vi "Drive Finish.vi"   [LabVIEW 2016]
uses:
  <vilib>/Rock Robotics/WPI/Ultrasonic/WPI_UltrasonicRangeUnits.ctl
  <vilib>/Rock Robotics/WPI/Utilities/WPI_GetSetVariantRefNum.vi
  <vilib>/Rock Robotics/WPI/Ultrasonic/WPI_SonarSRF04DigitalRefNum Registry Get.vi
  <vilib>/Rock Robotics/WPI/Ultrasonic/WPI_SonarSRF04DigitalClose.vi
types:
  T1 = typedef "WPI_UltrasonicRangeUnits.ctl" = enum16{"inches", "mm"}
  T2 = typedef "WPI_SolenoidDevRef.ctl" = cluster{"DevStatus":errorcluster, "Pneumatics Control Module":u8, "Forward Solenoid Channel":T3, "Reverse Solenoid Channel":T3}
  T3 = typedef "WPI_SolenoidChannel.ctl" = enum8{"Solenoid 0", "Solenoid 1", "Solenoid 2", "Solenoid 3", "Solenoid 4", "Solenoid 5", "Solenoid 6", "Solenoid 7", "Invalid"}
  T4 = typedef "WPI_JoystickDevRef.ctl" = cluster{"Device":T5}
  T5 = typedef "WPI_JoystickDeviceEnum.ctl" = enum16{"USB 0", "USB 1", "USB 2", "USB 3", "USB 4", "USB 5"}
  T6 = typedef "WPI_RobotDriveDevRef.ctl" = cluster{"DevStatus":errorcluster, "Motors[]":T7[], "Square Inputs":bool, "Max Output":dbl}
  T7 = typedef "WPI_MotorControlDeviceRef.ctl" = cluster{"DeviceStatus":errorcluster, "Type":T8, "PWM":cluster{"PWM Channel":T9, "DeadBand":T10}, "CAN":cluster{"Device Number":u8, "SetOutput VI Ref":variant, "GetOutput VI Ref":variant, "Enable VI Ref":variant, "Disable VI Ref":variant, "Data":variant}, "Invert":bool}
  T8 = typedef "WPI_MotorControlType.ctl" = enum16{"PWM", "CAN"}
  T9 = typedef "FPGA_DIOPWMChannel.ctl" = enum8{"PWM 0", "PWM 1", "PWM 2", "PWM 3", "PWM 4", "PWM 5", "PWM 6", "PWM 7", "PWM 8", "PWM 9", "PWM MXP 0", "PWM MXP 1", "PWM MXP 2", "PWM MXP 3", "PWM MXP 4", "PWM MXP 5", "PWM MXP 6", "PWM MXP 7", "PWM MXP 8", "PWM MXP 9", "Invalid"}
  T10 = typedef "WPI_PWMDeadband.ctl" = cluster{"Name":string, "maxPositivePwm":i32, "minPositivePwm":i32, "centerPwm":i32, "maxNegativePwm":i32, "minNegativePwm":i32, "angularRange":u16}
  T11 = typedef "WPI_CompressorDevRef.ctl" = cluster{"DevStatus":errorcluster, "Pneumatics Control Module":u8}
  T12 = typedef "WPI_EncoderDevRef.ctl" = cluster{"DevStatus":errorcluster, "EncoderIndex":T13, "CounterIndex":T14, "DistancePerCount":dbl, "Decoding Type":T15}
  T13 = typedef "FPGA_EncoderIdx.ctl" = enum8{"Enc 0", "Enc 1", "Enc 2", "Enc 3", "Enc 4", "Enc 5", "Enc 6", "Enc 7", "Invalid"}
  T14 = typedef "FPGA_CounterCtrSystemIndex.ctl" = enum8{"Ctr 0", "Ctr 1", "Ctr 2", "Ctr 3", "Ctr 4", "Ctr 5", "Ctr 6", "Ctr 7", "Invalid"}
  T15 = typedef "WPI_EncoderType.ctl" = enum16{"1x", "2x", "4x"}
  T16 = typedef "WPI_UltrasonicDeviceRef.ctl" = cluster{"DevStatus":errorcluster, "Ping Channel":T17, "Echo Channel":T17, "CntIndex":T14}
  T17 = typedef "FPGA_DIOChannel.ctl" = enum8{"DIO 0", "DIO 1", "DIO 2", "DIO 3", "DIO 4", "DIO 5", "DIO 6", "DIO 7", "DIO 8", "DIO 9", "DIO MXP 0", "DIO MXP 1", "DIO MXP 2", "DIO MXP 3", "DIO MXP 4", "DIO MXP 5", "DIO MXP 6", "DIO MXP 7", "DIO MXP 8", "DIO MXP 9", "DIO MXP 10", "DIO MXP 11", "DIO MXP 12", "DIO MXP 13", "DIO MXP 14", "DIO MXP 15", "SPI Port CS1", "SPI Port CS2", "SPI Port CS3", "SPI Port MISO", "SPI Port MOSI", "Invalid"}
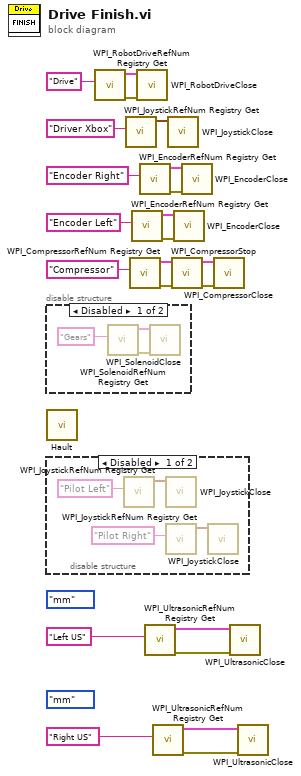
[diagram p0: block diagram]
diagram:
  (unwired) WPI_UltrasonicRangeUnits."mm" ("Range Units")
  (unwired) WPI_UltrasonicRangeUnits."mm" ("Range Units")
  n1 = disable-structure shown="Disabled" {
    frame Disabled {
      n2 = call <vilib>:"WPI_SolenoidRefNum Registry Get.vi"("refnum name"="Gears") -> ("error out"=w24:errorcluster, "SolenoidDevRef"=w25:T2)  [unwired: 9 in]
      n3 = call <vilib>:"WPI_SolenoidClose.vi"("error in (no error)"=w24, "SolenoidDevRef"=w25) -> ()  [unwired: 9 in, 1 out]
    }
    frame Enabled {
    }
  }
  n4 = call <vilib>:"Hault.vi"() -> ()  [unwired: 12 in]
  n5 = disable-structure shown="Disabled" {
    frame Disabled {
      n6 = call <vilib>:"WPI_JoystickRefNum Registry Get.vi"("refnum name"="Pilot Left") -> ("JoystickDevRef"=w28:T4)  [unwired: 9 in, 1 out]
      n7 = call <vilib>:"WPI_JoystickClose.vi"("JoystickDevRef"=w28) -> ()  [unwired: 11 in]
      n8 = call <vilib>:"WPI_JoystickRefNum Registry Get.vi"("refnum name"="Pilot Right") -> ("JoystickDevRef"=w27:T4)  [unwired: 9 in, 1 out]
      n9 = call <vilib>:"WPI_JoystickClose.vi"("JoystickDevRef"=w27) -> ()  [unwired: 11 in]
    }
    frame Enabled {
    }
  }
  n10 = call <vilib>:"WPI_RobotDriveRefNum Registry Get.vi"("refnum name"="Drive") -> ("error out"=w21:errorcluster, "RobotDriveDevRef"=w22:T6)  [unwired: 9 in]
  n11 = call <vilib>:"WPI_JoystickRefNum Registry Get.vi"("refnum name"="Driver Xbox") -> ("JoystickDevRef"=w19:T4)  [unwired: 9 in, 1 out]
  n12 = call <vilib>:"WPI_CompressorRefNum Registry Get.vi"("refnum name"="Compressor") -> ("error out"=w16:errorcluster, "CompressorDevRef"=w15:T11)  [unwired: 9 in]
  n13 = call <vilib>:"WPI_EncoderRefNum Registry Get.vi"("refnum name"="Encoder Left") -> ("error out"=w8:errorcluster, "EncoderDevRef"=w9:T12)  [unwired: 9 in]
  n14 = call <vilib>:"WPI_RobotDriveClose.vi"("error in (no error)"=w21, "RobotDriveDevRef"=w22) -> ()  [unwired: 9 in, 1 out]
  n15 = call <vilib>:"WPI_EncoderRefNum Registry Get.vi"("refnum name"="Encoder Right") -> ("error out"=w10:errorcluster, "EncoderDevRef"=w11:T12)  [unwired: 9 in]
  n16 = call-poly <vilib>:"WPI_UltrasonicRefNum Registry Get.vi"("refnum name"="Left US") -> ("error out"=w3:errorcluster, "SonarSRF04DevRef"=w2:T16)  [unwired: 9 in]
  n17 = call-poly <vilib>:"WPI_UltrasonicRefNum Registry Get.vi"("refnum name"="Right US") -> ("error out"=w5:errorcluster, "SonarSRF04DevRef"=w4:T16)  [unwired: 9 in]
  n18 = call <vilib>:"WPI_JoystickClose.vi"("JoystickDevRef"=w19) -> ()  [unwired: 11 in]
  n19 = call <vilib>:"WPI_CompressorStop.vi"("error in (no error)"=w16, "CompressorDevRef"=w15) -> ("error out"=w14:errorcluster, "CompressorDevRef"=w13:T11)  [unwired: 8 in]
  n20 = call <vilib>:"WPI_EncoderClose.vi"("error in (no error)"=w8, "EncoderDevRef"=w9) -> ()  [unwired: 9 in, 1 out]
  n21 = call <vilib>:"WPI_EncoderClose.vi"("error in (no error)"=w10, "EncoderDevRef"=w11) -> ()  [unwired: 9 in, 1 out]
  n22 = call <vilib>:"WPI_CompressorClose.vi"("error in (no error)"=w14, "CompressorDevRef"=w13) -> ()  [unwired: 9 in, 1 out]
  n23 = call-poly <vilib>:"WPI_UltrasonicClose.vi"("error in (no error)"=w3, "SonarSRF04DevRef"=w2) -> ()  [unwired: 9 in, 1 out]
  n24 = call-poly <vilib>:"WPI_UltrasonicClose.vi"("error in (no error)"=w5, "SonarSRF04DevRef"=w4) -> ()  [unwired: 9 in, 1 out]
